vi "dipose.vi"(8 "error in (no error)":errorcluster, 11 "TCP Socket Server in":refnum<class "TCP Socket Server.lvclass">) -> (0 "error out":errorcluster)   [LabVIEW 2019, in "TCP Socket Server.lvclass"]
uses:
  TCP Socket Server.lvclass
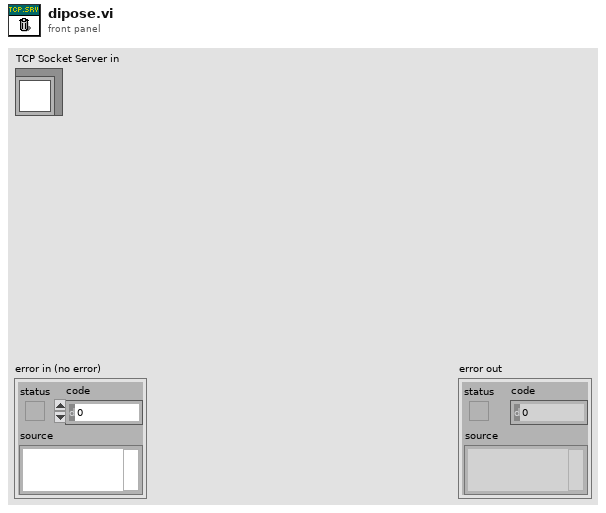
[diagram p1: front panel]
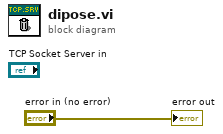
[diagram p0: block diagram]
diagram:
  "error out" <- "error in (no error)"
